vi "Visa_Write read_UI GETPORT.vi"(0 "Serial Device in":refnum<class "Serial Device.lvclass">, 1 "VISA resource name":refnum<visa-resource-name>, 2 "Command to Send":string, 3 "Expected Response":string, 4 "Buttons":bool[](array[boolean]), 5 "error in (no error)":errorcluster) -> (14 "Serial Device out":refnum<class "Serial Device.lvclass">, 15 "VISA Refnum out":refnum<visa-resource-name>, 16 "Expected Response out":string, 17 "Port":string, 19 "error out":errorcluster)   [LabVIEW 2020, in "Serial Device.lvclass"]
uses:
  Serial Device.lvclass
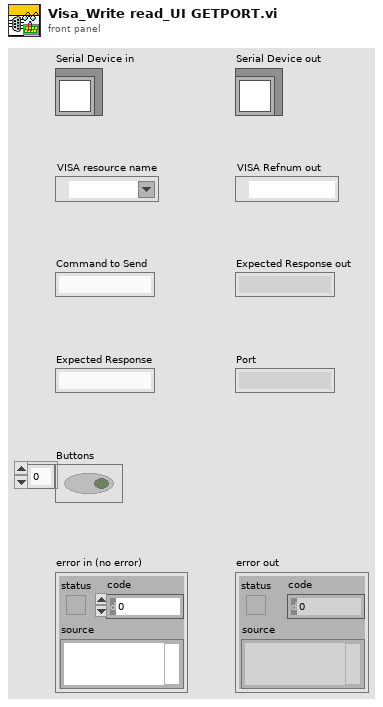
[diagram p1: front panel]
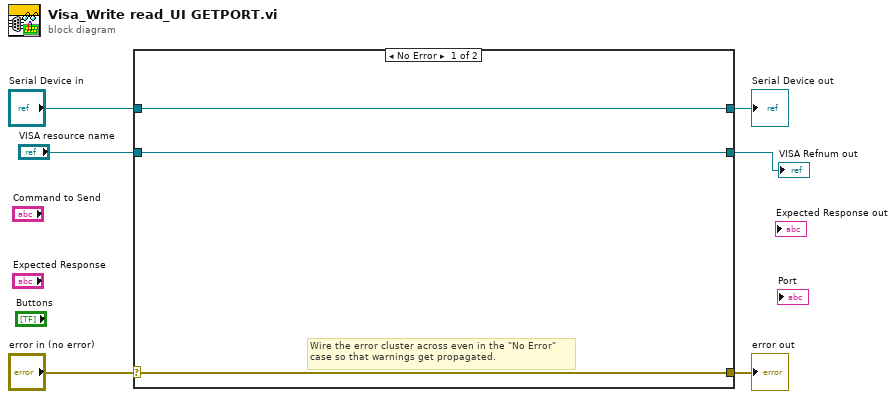
[diagram p0: block diagram]
diagram:
  n1 = case shown="No Error" "error in (no error)" {
    selector: "error in (no error)" -> [w8 w11]
    tunnel: [w8 w11] -> w5
    tunnel: [w9 w10] -> w3
    tunnel: "Serial Device in" -> [w9 w10]
    tunnel: [w7 _] -> w2
    tunnel: "VISA resource name" -> [w7 _]
    frame No Error {
      # "Wire the error cluster across even in the \"No Error\"\ncase so that warnings get propagated."
    }
    frame Error {
    }
  }
  "error out" <- w5
  "Serial Device out" <- w3
  "VISA Refnum out" <- w2
